vi "prepDO_img.vi"() -> ()   [LabVIEW 2015]
uses:
  <vilib>/DAQmx/write.llb/DAQmx Write (Digital 1D Wfm NChan NSamp).vi
  waveforms/usedDOindepofwf.vi
  Objects/waveformsDObuffer.vi
  <vilib>/DAQmx/create/channels.llb/DAQmx Create Channel (DO-Digital Output).vi
  <vilib>/DAQmx/configure/timing.llb/DAQmx Timing (Sample Clock).vi
  <vilib>/Waveform/DWDTOps.llb/DWDT Uncompress Digital.vi
  <vilib>/DAQmx/miscellaneous.llb/DAQmx Fill In Error Info.vi
panel:
  in  "error in":errorcluster
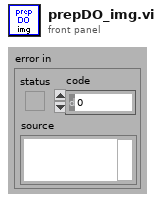
[diagram p1: front panel]
types:
  T1 = typedef "XYZStage.lvlib/XYZStage Configuration.ctl" = cluster{"VISA resource name":refnum<visa-resource-name>, "Timeout (3sec)":u32}
  T2 = cluster{"StageS":i32, "StageL":i32, "currmeas data dir":path, "image OD":u16, "contour OD":u16, "point OD":u16, "AOlines":tag[], "AIlines":tag[], "CI lines":tag[], "DO lines":tag[], "AO names":string[], "CI names":string[], "AI names":string[], "DO names":string[], "CIextensions":string[], "AIextensions":string[], "Voltage to Ygalvo":i32, "Voltage to Xgalvo":i32, "Voltage to patch":i32, "640 shutter":i32, "2P shutter":i32, "LT timestamp":u32, "Vp":i32, "Ip":i32, "camera trigger":i32, "master data dir":path, "voltage to Zpos":i32, "Vto2P":i32, "640 AO":i32, "488 AO":i32, "532 AO":i32, "640TTL":u32, "488TTL":u32, "532TTL":u32, "Device 1 sampleclock out":tag, "Device 1 Starttrigger out":tag, "Device 2 sampleclock in":tag, "Device 2 StartTrigger in ":tag, "2PODTTL":u32, "488 shutter":u32, "LCVR red":u32, "LCVR blue":u32, "Sutter Stage Config":T1}
  T3 = typedef "LVRectTypeDef.ctl" = cluster{"Left":i16, "Top":i16, "Right":i16, "Bottom":i16}
  T4 = cluster{"Xpixels":i32, "Vxminref":dbl, "Vxmaxref":dbl, "P":dbl, "Ypixels":i32, "Vyminref":dbl, "Vymaxref":dbl, "srate":sgl, "sAOxy":i32, "timeout":dbl, "type":string, "date":string, "time":string, "Colormap":u16, "Drawing Mode":u16, "Scanning Mode":u16, "square pixels":bool, "square matrix":bool, "Xpixels Img":i32, "Vx-min Img":dbl, "VX-max Img":dbl, "Ypixels Img":i32, "Vy-min Img":dbl, "Vy-max Img ":dbl, "Angle Img":dbl, "autoshutter":bool, "finite":bool, "cont":bool, "wavdet":bool, "measpoints":i32, "avpp":i32, "bufferAO":i32, "bufferAI":i32, "starttick":u32, "waveform":path, "Vx-ref":dbl, "Vy-ref":dbl, "refreshrate":dbl, "refreshbuffer":i32, "tt_cycles":i32, "motorref":refnum<k7>, "mirrorswitch":refnum<k7>, "sample mode":i32, "maxbufferAI":i32, "srateAODO":sgl, "bin":sgl, "Pel":sgl, "Angle draw":dbl, "srate Img":sgl, "ROIimg_plotbounds":T3, "auto OD":bool, "ODfilt":u16, "aAI":i32[], "aCI":i32[], "aAO":u32[], "aDO":u32[], "refwfsize":dbl, "Lifetime":bool, "Vz-Img":dbl, "Vz-ref":dbl, "Vz-reset":dbl, "AIoverride":bool, "aAS":u32[], "XYZstart":dbl[]}
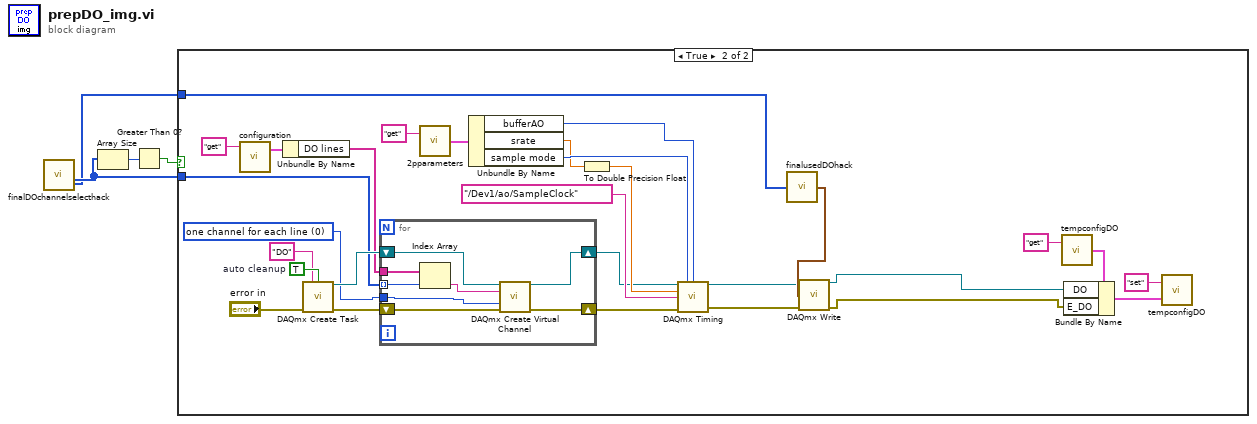
[diagram p0: block diagram]
diagram:
  n1 = call "finalDOchannelselecthack.vi"() -> ("usedDO"=w2:u32[], "presorted indices"=w1:u32[])  [unwired: 1 in]
  n2 = Array Size(array=w2) -> (size(s)=w3:i32)
  n3 = Greater Than 0?(x=w3) -> (x > 0?=w4:bool)
  n4 = case shown="True" w4 {
    tunnel: w2 -> [_ w21]
    tunnel: w1 -> [_ w6]
    frame False {
    }
    frame True {
      w12 = 0 items=["one channel for each line", "one channel for all lines"] ("line grouping")
      w32 = TRUE  # auto cleanup
      n5 = call "configuration.vi"("command"="get") -> ("config out"=w14:T2)  [unwired: 2 in, 1 out]
      n6 = Unbundle By Name(w14) -> ("DO lines"=w13:tag[])
      n7 = call <vilib>:"DAQmx Create Task.vi"("new task name"="DO", "auto cleanup"=w32, "error in"="error in") -> ("task out"=w33:refnum<k21>, "error out"=w31:errorcluster)  [unwired: 11 in]
      n8 = for {
        shift-right: [w36] -> w24
        shift-left: w31 -> [w40]
        tunnel: w21 -> [w39] mode=indexing
        shift-right: [w37] -> w25
        shift-left: w33 -> [w41]
        tunnel: w13 -> [w35]
        tunnel: w12 -> [w34]
        n9 = Index Array(array=w35, index=w39) -> (element=w38:tag)
        n10 = call-poly <vilib>:"DAQmx Create Virtual Channel.vi"("task in"=w41, "lines"=w38, "line grouping"=w34, "error in"=w40) -> ("task out"=w37:refnum<k21>, "error out"=w36:errorcluster)  [unwired: 10 in]
      }
      n11 = call "2pparameters.vi"("command"="get") -> ("params out"=w29:T4)  [unwired: 1 in]
      n12 = Unbundle By Name(w29) -> ("bufferAO"=w23:i32, "srate"=w16:sgl, "sample mode"=w22:i32)
      n13 = To Double Precision Float(number=w16) -> (double precision float=w27:dbl)
      n14 = call-poly <vilib>:"DAQmx Timing.vi"("task/channels in"=w25, "sample mode"=w22, "samples per channel"=w23, "rate"=w27, "source"=tag "/Dev1/ao/SampleClock", "error in"=w24) -> ("task out"=w10:refnum<k21>, "error out"=w9:errorcluster)  [unwired: 1 in, 7 out]
      n15 = call "finalusedDOhack.vi"("presorted indices"=w6) -> ("DO"=w11:digitalwaveform[])
      n16 = call-poly <vilib>:"DAQmx Write.vi"("task/channels in"=w10, "data"=w11, "error in"=w9) -> ("task out"=w8:refnum<k21>, "error out"=w7:errorcluster)  [unwired: 10 in, 1 out]
      n17 = call "tempconfigDO.vi"("command"="get") -> ("Temp Config out"=w19:cluster{"DO":refnum<k21>, "E_DO":errorcluster})  [unwired: 1 in]
      n18 = Bundle By Name(cluster=w19, "DO"=w8, "E_DO"=w7) -> (w17:cluster{"DO":refnum<k21>, "E_DO":errorcluster})
      n19 = call "tempconfigDO.vi"("Temp Config in"=w17, "command"="set") -> ()  [unwired: 1 out]
    }
  }
